vi "Stop.vi"(8 "error in (no error)":errorcluster, 11 "ConsoleOutput in":refnum<class "ConsoleOutput.lvclass">) -> (0 "error out":errorcluster, 3 "ConsoleOutput out":refnum<class "ConsoleOutput.lvclass">)   [LabVIEW 2020, in "ConsoleOutput.lvclass"]
uses:
  ConsoleOutput.lvclass
  ConsoleOutput.lvclass/ConsoleOutput.ctl
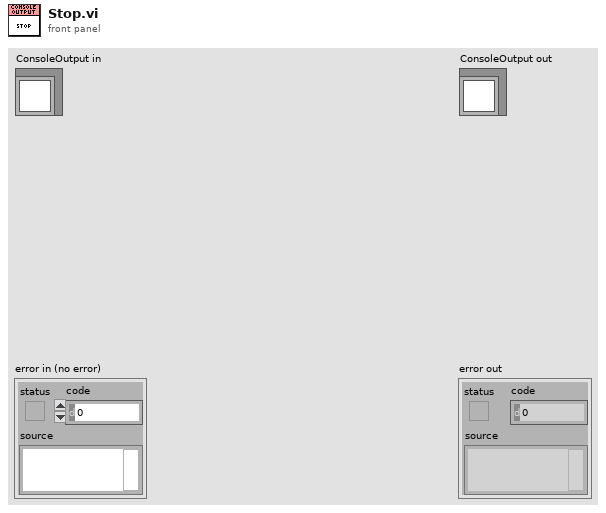
[diagram p1: front panel]
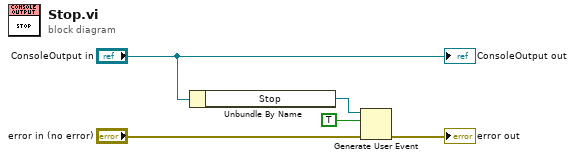
[diagram p0: block diagram]
diagram:
  n1 = Unbundle By Name("ConsoleOutput in") -> ("Stop"=w2:refnum<user-event>)
  n2 = Generate User Event(user event=w2, event data cluster=TRUE ("event data"), error in="error in (no error)") -> (error out=→"error out":errorcluster)  [unwired: 1 in, 1 out]
  "ConsoleOutput out" <- "ConsoleOutput in"
